vi "Is Non-Special Pattern Char.vi"(7 "Value":string, 8 "Constructor String Parser":T1, 9 "Index":i32) -> (2 "Non-Special Pattern Char?":bool)   [LabVIEW 2020, in "Stream.lvlib" / "URLPattern.lvclass"]
uses:
  URLPattern.lvclass
  Constructor String Parser.ctl
  Token.ctl
  Token Type.ctl
  URL Pattern Init.ctl
  Parser State.ctl
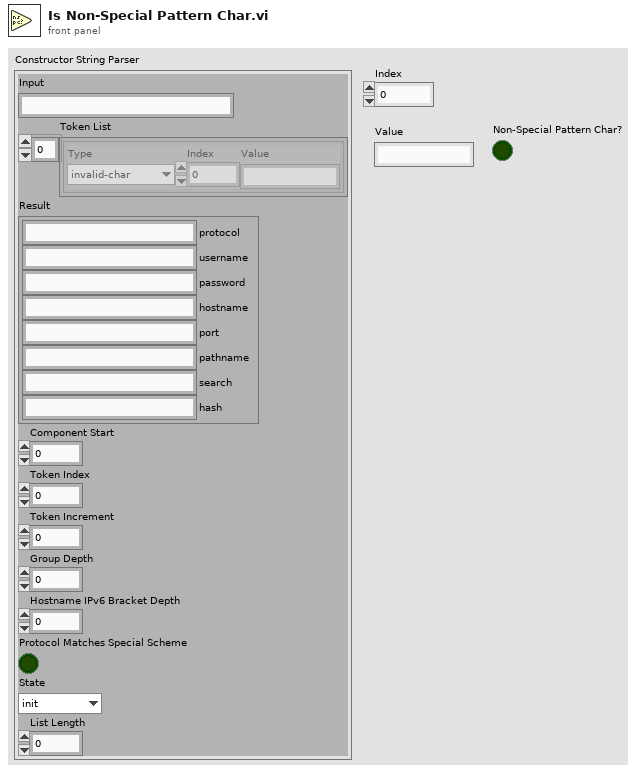
[diagram p1: front panel]
types:
  T1 = typedef "Stream.lvlib/URLPattern.lvclass/Constructor String Parser.ctl" = cluster{"Input":string, "Token List":T2[], "Result":T4, "Component Start":i32, "Token Index":i32, "Token Increment":i32, "Group Depth":i32, "Hostname IPv6 Bracket Depth":i32, "Protocol Matches Special Scheme":bool, "State":T5, "List Length":i32}
  T2 = typedef "Stream.lvlib/URLPattern.lvclass/Token.ctl" = cluster{"Type":T3, "Index":i32, "Value":string}
  T3 = typedef "Stream.lvlib/URLPattern.lvclass/Token Type.ctl" = enum16{"invalid-char", "open", "close", "regexp", "name", "char", "escaped-char", "other-modifier", "asterisk", "end"}
  T4 = typedef "Stream.lvlib/URLPattern.lvclass/URL Pattern Init.ctl" = cluster{"protocol":string, "username":string, "password":string, "hostname":string, "port":string, "pathname":string, "search":string, "hash":string}
  T5 = typedef "Stream.lvlib/URLPattern.lvclass/Parser State.ctl" = enum16{"init", "protocol", "authority", "username", "password", "hostname", "port", "pathname", "search", "hash", "done"}
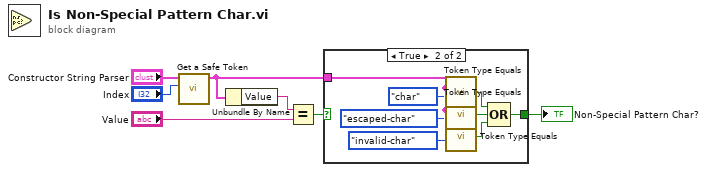
[diagram p0: block diagram]
diagram:
  n1 = call "Get a Safe Token.vi"("Index"="Index", "Constructor String Parser"="Constructor String Parser") -> ("Token"=w1:T2)  [unwired: 8 in, 1 out]
  n2 = Unbundle By Name(w1) -> ("Value"=w4:string)
  n3 = Equal?(x=w4, y="Value") -> (x = y?=w3:bool)
  n4 = case shown="True" w3 {
    selector: w3 -> [w8 _]
    tunnel: [w8 w9] -> w2
    tunnel: w1 -> [_ w16]
    frame False {
    }
    frame True {
      n5 = call "Token Type Equals.vi"("Type"=Token_Type."char", "Token"=w16) -> ("Type Equals?"=w11:bool)  [unwired: 2 in]
      n6 = call "Token Type Equals.vi"("Type"=Token_Type."escaped-char", "Token"=w16) -> ("Type Equals?"=w12:bool)  [unwired: 2 in]
      n7 = call "Token Type Equals.vi"("Type"=Token_Type."invalid-char", "Token"=w16) -> ("Type Equals?"=w10:bool)  [unwired: 2 in]
      n8 = Compound Arithmetic op=OR(w11, w12, w10) -> (w9:bool)
    }
  }
  "Non-Special Pattern Char?" <- w2
